vi "XML429_Database_LoadConfig.vi"(0 "FilePath":path, 11 "Error in":errorcluster) -> (4 "ConfigHandle":refnum<k20>, 15 "Error out":errorcluster)   [LabVIEW 2015, in "AIT 429 System Explorer.lvlib"]
doc: "XML429_Database_LoadConfig"
uses:
  <vilib>/xml/Load XML File.vi
  AIT 429 System Explorer.lvlib
  <vilib>/xml/NI_XML.lvlib
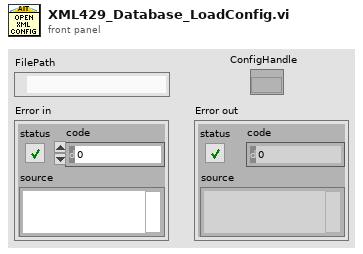
[diagram p1: front panel]
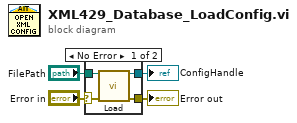
[diagram p0: block diagram]
diagram:
  n1 = case shown="No Error" "Error in" {
    selector: "Error in" -> [w8 w9]
    tunnel: [w7 w9] -> w3
    tunnel: "FilePath" -> [w6 _]
    tunnel: [w5 _] -> w1
    frame No Error {
      n2 = call-poly <vilib>:"Load.vi"("path to XML document"=w6, "error in (no error)"=w8) -> ("DOM document out"=w5:refnum<k20>, "error out"=w7:errorcluster)  [unwired: 11 in, 1 out]
    }
    frame Error {
    }
  }
  "Error out" <- w3
  "ConfigHandle" <- w1
